vi "ndipolaris Initialize.vi"(7 "Serial Configuration":T1={"Baud Rate (9600)"=9600, "Flow Control (0:None)"=0, "Parity"=0, "Data Bits"=8, "Stop Bits"=10} {"Stop Bits" items=["1.0"=10, "2.0"=20]; "Parity" items=["None", "Odd", "Even"]; "Flow Control (0:None)" items=["None", "XON/XOFF"]; "Baud Rate (9600)" items=["9600"=9600, "14.4k"=14400, "19.2k"=19200, "38.4k"=38400, "57.6k "=57600, "115.2k"=115200]}, 8 "error in (no error)":errorcluster, 9 "Reset? (T: Yes)":bool=TRUE, 11 "VISA resource name":refnum<visa-resource-name>="COM1") -> (0 "error out":errorcluster, 3 "VISA resource name out":refnum<visa-resource-name>)   [LabVIEW 2013]
doc: "This VI opens a VISA session for the VISA resource name specified. You can optionally reset the instrument by setting the front panel reset control. You must run this VI before using any of the instrument driver VIs for this instrument.\n\nNotes:\n\n(1) This instrument driver supports serial communication. If problems are encountered when using serial communication, it is recommended to try using the 9600 baud rate. \n\n(2) If you do wish to use the serial interface, set the serial settings on the instrument to be the same as the serial settings on the block diagram and in Measurement & Automation Explorer."
panel:
  # "© 2004 National Instruments Corporation.  ALL RIGHTS RESERVED."
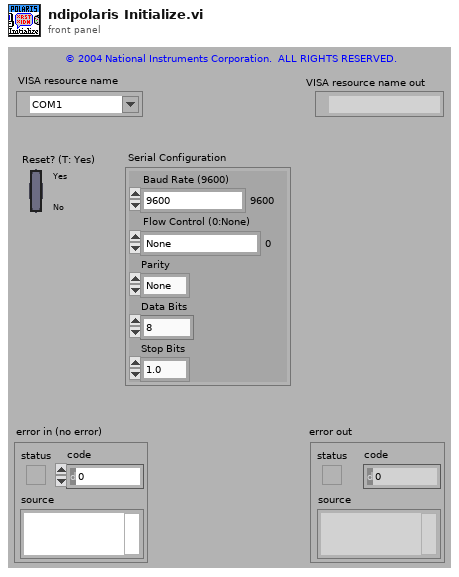
[diagram p1: front panel]
types:
  T1 = cluster{"Baud Rate (9600)":u32, "Flow Control (0:None)":u16, "Parity":u16, "Data Bits":u16, "Stop Bits":u16}
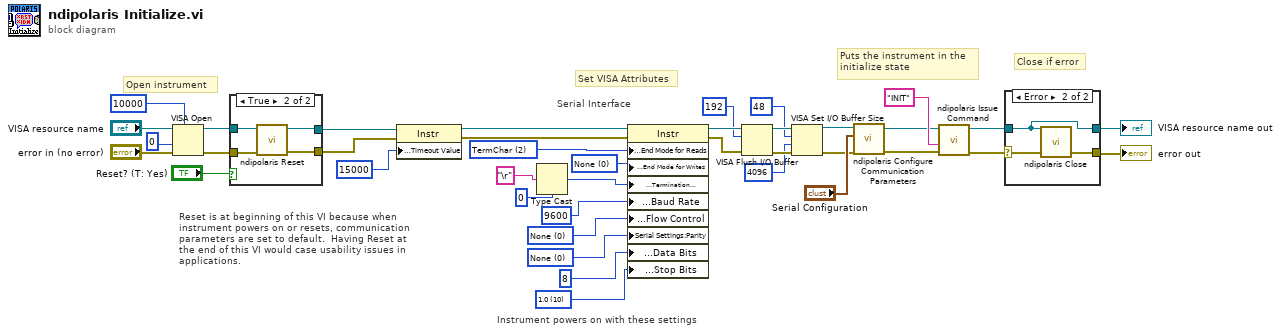
[diagram p0: block diagram]
diagram:
  w16 = u16 10 items=["1.0"=10, "1.5"=15, "2.0"=20] ("Serial Settings:Serial Stop Bits")
  w17 = u16 0 items=["None", "Odd", "Even", "Mark", "Space"] ("Serial Settings:Serial Parity")
  w18 = u16 0 items=["None", "XON/XOFF", "RTS/CTS", "XON/XOFF & RTS/CTS", "DTR/DSR", "XON/XOFF & DTR/DSR"] ("Serial Settings:Serial Flow Control")
  w23 = u16 0 items=["None", "LastBit", "TermChar", "Break"] ("Serial Settings:Serial End Mode for Writes")
  w24 = u16 2 items=["None", "LastBit", "TermChar"] ("Serial Settings:Serial End Mode for Reads")
  # "Reset is at beginning of this VI because when\ninstrument powers on or resets, communication \nparameters are set to default.  Having Reset at\nthe end of this VI would case usability issues in\napplications."
  # "Puts the instrument in the\ninitialize state"
  # "Close if error"
  # "Instrument powers on with these settings"
  # "Serial Interface"
  # "Set VISA Attributes"
  # "Open instrument"
  n1 = VISA Open(timeout (0)=u32 10000 ("VISA Open timeout (0)"), access mode=u32 0, error in (no error)="error in (no error)", VISA resource name="VISA resource name") -> (VISA resource name=w2:refnum<visa-resource-name>, error out=w1:errorcluster)  [unwired: 1 in]
  n2 = case shown="True" "Reset? (T: Yes)" {
    tunnel: [w41 w45] -> w4
    tunnel: [w40 w44] -> w5
    tunnel: w2 -> [w41 w43]
    tunnel: w1 -> [w40 w42]
    frame False {
    }
    frame True {
      n3 = call <instrlib>:"ndipolaris Reset.vi"("error in (no error)"=w42, "VISA resource name"=w43) -> ("error out"=w44:errorcluster, "VISA resource out"=w45:refnum<visa-resource-name>)  [unwired: 8 in]
    }
  }
  n4 = property class="Instr"(reference=w4, error in=w5, "General Settings:Timeout Value"=u32 15000) -> (reference out=w38:refnum<visa-resource-name>, error out=w39:errorcluster)
  n5 = Type Cast(type=u8 0, x="\r") -> (*(type *) &x=w25:u8)
  n6 = property class="Instr"(reference=w38, error in=w39, "Serial Settings:End Mode for Reads"=w24, "Serial Settings:End Mode for Writes"=w23, "Message Based Settings:Termination Character"=w25, "Serial Settings:Baud Rate"=u32 9600 ("Serial Settings:Serial Baud Rate"), "Serial Settings:Flow Control"=w18, "Serial Settings:Parity"=w17, "Serial Settings:Data Bits"=u16 8 ("Serial Settings:Serial Data Bits"), "Serial Settings:Stop Bits"=w16) -> (reference out=w30:refnum<visa-resource-name>, error out=w32:errorcluster)
  n7 = VISA Flush I/O Buffer(VISA resource name=w30, mask (16)=u16 192, error in (no error)=w32) -> (VISA resource name out=w33:refnum<visa-resource-name>, error out=w31:errorcluster)
  n8 = VISA Set I/O Buffer Size(VISA resource name=w33, mask (16)=u16 48, size (4096)=u32 4096 ("size (0)"), error in (no error)=w31) -> (VISA resource name out=w14:refnum<visa-resource-name>, error out=w13:errorcluster)
  n9 = call <instrlib>:"ndipolaris Configure Communication Parameters.vi"("error in (no error)"=w13, "Serial Configuration"="Serial Configuration", "VISA resource name"=w14) -> ("error out"=w12:errorcluster, "VISA resource out"=w11:refnum<visa-resource-name>)  [unwired: 7 in]
  n10 = call <instrlib>:"ndipolaris Issue Command.vi"("error in (no error)"=w12, "Write Buffer"="INIT" ("write buffer"), "VISA resource name"=w11) -> ("error out"=w6:errorcluster, "VISA resource out"=w20:refnum<visa-resource-name>)  [unwired: 6 in, 1 out]
  n11 = case shown="Error" w6 {
    selector: w6 -> [w46 w48]
    tunnel: w20 -> [w47 w49]
    tunnel: [w47 w49] -> w36
    tunnel: [w46 w50] -> w35
    frame No Error {
    }
    frame Error {
      n12 = call <instrlib>:"ndipolaris Close.vi"("error in (no error)"=w48, "VISA resource name"=w49) -> ("error out"=w50:errorcluster)  [unwired: 9 in]
    }
  }
  "VISA resource name out" <- w36
  "error out" <- w35
